vi "Read Open.vi"(8 "error in (no error)":errorcluster, 11 "dir in":refnum<class "dir.lvclass">) -> (0 "error out":errorcluster, 2 "Open":bool, 3 "dir out":refnum<class "dir.lvclass">)   [LabVIEW 2023, in "d7.lvlib" / "dir.lvclass"]
uses:
  dir.lvclass
  dir.lvclass/dir.ctl
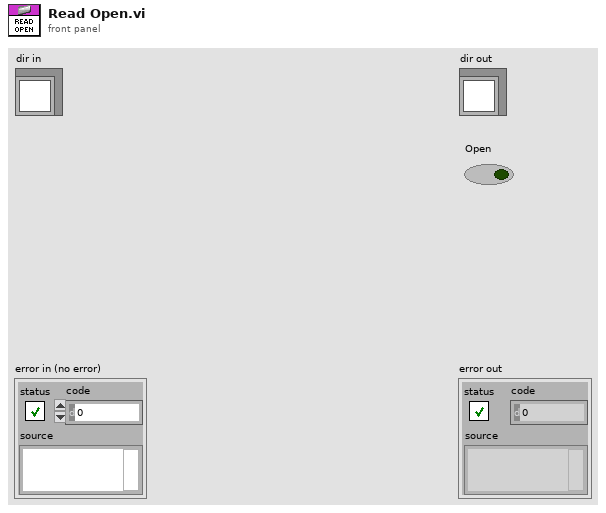
[diagram p1: front panel]
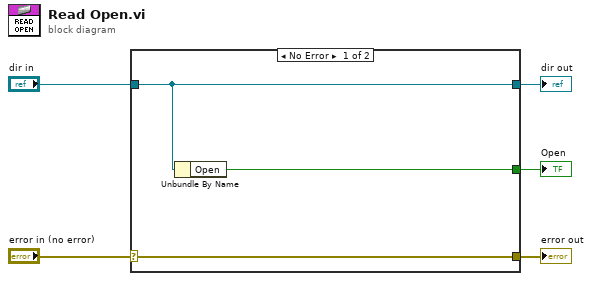
[diagram p0: block diagram]
diagram:
  n1 = case shown="No Error" "error in (no error)" {
    selector: "error in (no error)" -> [w8 w9]
    tunnel: [w8 w9] -> w4
    tunnel: [w7 w10] -> w2
    tunnel: "dir in" -> [w7 w10]
    tunnel: [w6 _] -> w1
    frame No Error {
      n2 = Unbundle By Name(w7) -> ("Open"=w6:bool)
    }
    frame Error {
    }
  }
  "error out" <- w4
  "dir out" <- w2
  "Open" <- w1
